vi "TIO Access Module Run.vi"(5 "Notification Prefix":string="Default", 8 "error in (no error)":errorcluster, 11 "TS Connection":T1={"Type"=enum."TCP", "Serial"="serial:///dev/cu.usbserial-00000", "TCP"=refnum, "Timeout"=500}) -> ()   [LabVIEW 2017]
uses:
  <vilib>/Utility/error.llb/Clear Errors.vi
  <instrlib>/tio-labview/TIO Library/Socket/TIO Stream Write.vi
  <instrlib>/tio-labview/TIO Library/RPC/RPC Helpers/TIO RPC Form Request.vi
  <instrlib>/tio-labview/TIO Library/Socket/Helpers/TIO SLIP Serial Write.vi
  <instrlib>/tio-labview/TIO Library/Socket/Helpers/TIO Form Packet.vi
  <instrlib>/tio-labview/TIO Library/Socket/Helpers/TIO SLIP Encode.vi
  <instrlib>/tio-labview/TIO Library/Socket/Helpers/TIO Serial Checksum CRC32.vi
panel:
  out "Kill":bool=TRUE
  out "Last Log":string
  out "Last PUB":string
  out "Last REQ":string
  # "TIO Proxy Run"
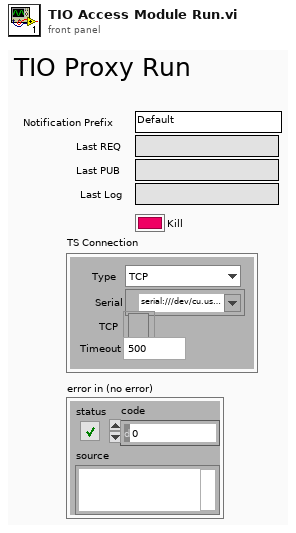
[diagram p1: front panel]
types:
  T1 = cluster{"Type":enum16{"TCP", "Serial"}, "Serial":refnum<visa-resource-name>, "TCP":refnum<k5>, "Timeout":u32}
  T2 = enum16{"big-endian, network order", "native, host order", "little-endian"}
  T3 = cluster{"Stream Description":cluster{"Stream ID":u16, "Data Type":u8, "Channels":u8, "Restart ID":u16, "Start timestamp (s)":dbl, "Sample counter":u64, "Period (s)":dbl, "Flags":u8, "Timestamp type":u8, "Name":string, "Last sample number":u64, "Last Restart ID":u16, "Version":u16, "Sample Size":u16}, "Sample #":u32, "Raw Data":string}
  T4 = cluster{"Stream ID":u16, "Data Type":u8, "Channels":u8, "Restart ID":u16, "Start timestamp (s)":dbl, "Sample counter":u64, "Period (s)":dbl, "Flags":u8, "Timestamp type":u8, "Name":string, "Last sample number":u64, "Last Restart ID":u16, "Version":u16, "Sample Size":u16}
  T5 = cluster{"Stream ID":u16, "Data Type":u8, "Channels":u8, "Restart ID":u16, "Start timestamp (s)":dbl, "Sample counter":u64, "Period (s)":dbl, "Flags":u8, "Timestamp type":u8, "Name":string, "Last sample number":u64, "Last Restart ID":u16, "Version":u16, "Sample Size":u16}[]
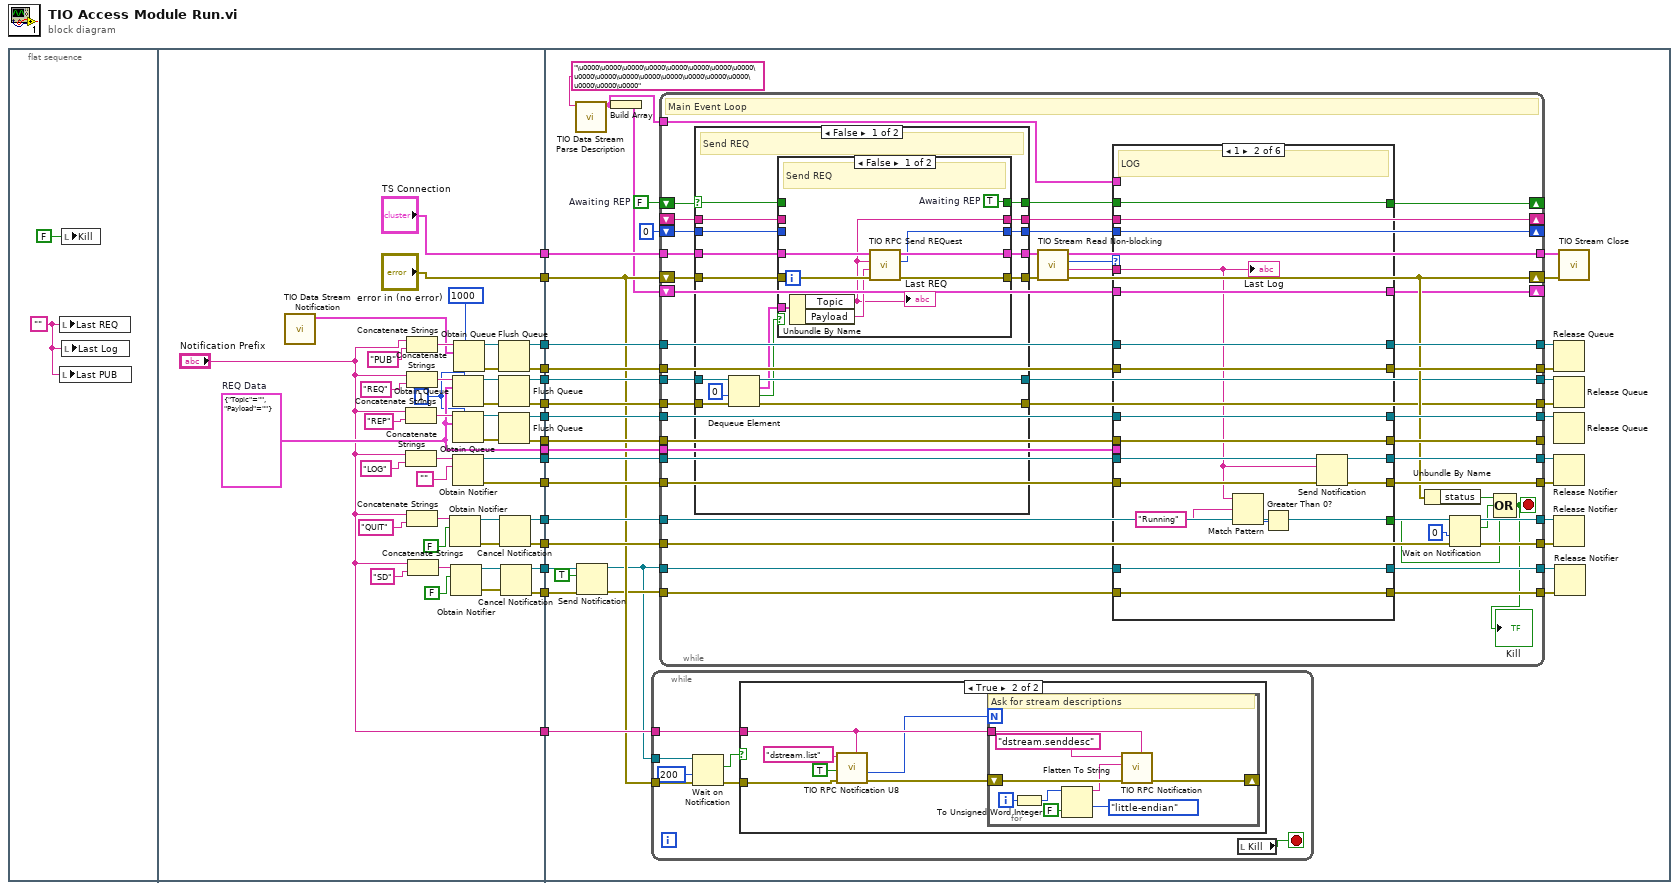
[diagram p0: block diagram]
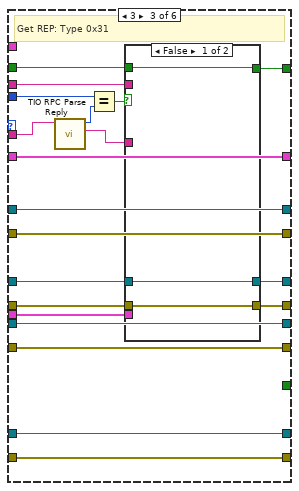
[diagram p4: hidden frame]
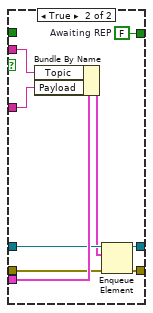
[diagram p5: hidden frame]
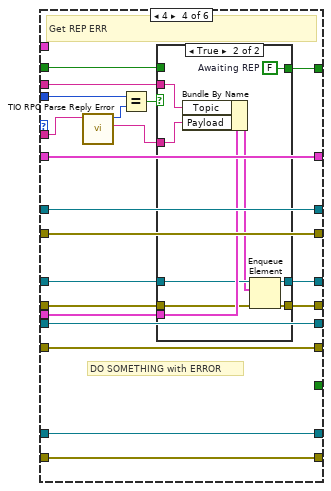
[diagram p6: hidden frame]
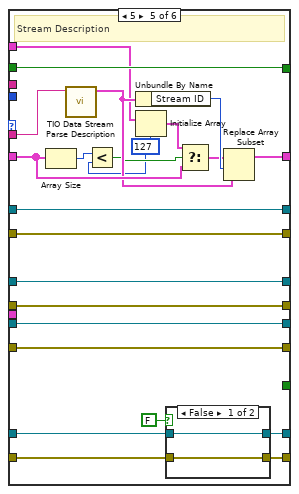
[diagram p8: hidden frame]
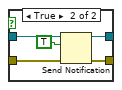
[diagram p9: hidden frame]
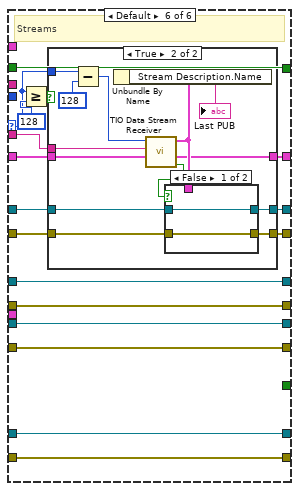
[diagram p10: hidden frame]
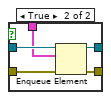
[diagram p12: hidden frame]
diagram:
  n1 = flat-sequence {
    tunnel: [w49] -> w16
    tunnel: ["Notification Prefix"] -> w15
    tunnel: ["TS Connection"] -> w14
    tunnel: ["error in (no error)"] -> w13
    tunnel: [w48] -> w12
    tunnel: [w38] -> w11
    tunnel: [w36] -> w10
    tunnel: [w35] -> w9
    tunnel: [w34] -> w8
    tunnel: [w40] -> w7
    tunnel: [w30] -> w6
    tunnel: [w29] -> w5
    tunnel: [w47] -> w4
    tunnel: [w46] -> w3
    tunnel: [w22] -> w2
    tunnel: [w21] -> w1
    tunnel: w16 -> [w92]
    tunnel: w15 -> [w80]
    tunnel: w14 -> [w91]
    tunnel: w13 -> [w79]
    tunnel: w12 -> [w90]
    tunnel: w11 -> [w89]
    tunnel: w10 -> [w88]
    tunnel: w9 -> [w87]
    tunnel: w8 -> [w86]
    tunnel: w7 -> [w85]
    tunnel: w6 -> [w84]
    tunnel: w5 -> [w83]
    tunnel: w4 -> [w82]
    tunnel: w3 -> [w81]
    tunnel: w2 -> [w71]
    tunnel: w1 -> [w70]
    frame #0 {
      w18 = ""
      n2 = local write "Last REQ"(w18) -> ()
      n3 = local write "Last PUB"(w18) -> ()
      n4 = local write "Kill"(FALSE ("Running")) -> ()
      n5 = local write "Last Log"(w18) -> ()
    }
    frame #1 {
      w33 = 1 ("max queue size (-1, unlimited)")
      w40 = cluster{"Topic":string, "Payload":string} {"Topic"="", "Payload"=""}  # REQ Data
      n6 = call <instrlib>:"TIO Data Stream Notification.vi"() -> ("Data Stream Notification"=w45:T3)  [unwired: 11 in]
      n7 = Concatenate Strings("Notification Prefix", "REP" ("name (unnamed)")) -> (w41:string)
      n8 = Concatenate Strings("Notification Prefix", "LOG" ("name (unnamed)")) -> (w32:string)
      n9 = Concatenate Strings("Notification Prefix", "PUB" ("name (unnamed)")) -> (w56:string)
      n10 = Concatenate Strings("Notification Prefix", "REQ" ("name (unnamed)")) -> (w42:string)
      n11 = Concatenate Strings("Notification Prefix", "QUIT" ("name (unnamed)")) -> (w52:string)
      n12 = Concatenate Strings("Notification Prefix", "SD" ("name (unnamed)")) -> (w26:string)
      n13 = Obtain Notifier(name (unnamed)=w52, notification data type=FALSE ("Connected")) -> (notifier out=w59:refnum<notifier>, error out=w60:errorcluster)  [unwired: 2 in, 1 out]
      n14 = Obtain Notifier(name (unnamed)=w26, notification data type=FALSE ("Connected")) -> (notifier out=w25:refnum<notifier>, error out=w24:errorcluster)  [unwired: 2 in, 1 out]
      n15 = Obtain Queue(max queue size (-1, unlimited)=w33, name (unnamed)=w42, element data type=w40) -> (queue out=w39:refnum<queue>, error out=w37:errorcluster)  [unwired: 2 in, 1 out]
      n16 = Obtain Queue(max queue size (-1, unlimited)=w33, name (unnamed)=w41, element data type=w40) -> (queue out=w44:refnum<queue>, error out=w43:errorcluster)  [unwired: 2 in, 1 out]
      n17 = Obtain Notifier(name (unnamed)=w32, notification data type="") -> (notifier out=w30:refnum<notifier>, error out=w29:errorcluster)  [unwired: 2 in, 1 out]
      n18 = Obtain Queue(max queue size (-1, unlimited)=1000, name (unnamed)=w56, element data type=w45) -> (queue out=w57:refnum<queue>, error out=w58:errorcluster)  [unwired: 2 in, 1 out]
      n19 = Flush Queue(queue=w57, error in (no error)=w58) -> (queue out=w49:refnum<queue>, error out=w48:errorcluster)  [unwired: 1 out]
      n20 = Flush Queue(queue=w39, error in (no error)=w37) -> (queue out=w38:refnum<queue>, error out=w36:errorcluster)  [unwired: 1 out]
      n21 = Flush Queue(queue=w44, error in (no error)=w43) -> (queue out=w35:refnum<queue>, error out=w34:errorcluster)  [unwired: 1 out]
      n22 = Cancel Notification(0:w59, 3:w60) -> (8:w47:refnum<notifier>, 11:w46:errorcluster)  [unwired: 1 out]
      n23 = Cancel Notification(0:w25, 3:w24) -> (8:w22:refnum<notifier>, 11:w21:errorcluster)  [unwired: 1 out]
    }
    frame #2 {
      w72 = FALSE  # Awaiting REP
      n24 = call <instrlib>:"TIO Data Stream Parse Description.vi"("Raw Stream Description"="\u0000\u0000\u0000\u0000\u0000\u0000\u0000\u0000\u0000\u0000\u0000\u0000\u0000\u0000\u0000\u0000\u0000\u0000\u0000") -> ("Stream Description"=w63:T4)  [unwired: 10 in]
      n25 = Send Notification(notification=TRUE, notifier=w71, error in (no error)=w70) -> (notifier out=w66:refnum<notifier>, error out=w69:errorcluster)
      n26 = Build Array(w63) -> (w78:T5)
      n27 = while {
        tunnel: w80 -> [w106]
        tunnel: w79 -> [w105]
        tunnel: w66 -> [w103]
        stop <- w102 stop-if-true
        n28 = Wait on Notification(notifier=w103, timeout in ms (-1)=200, error in (no error)=w105) -> (notification=w100:bool, error out=w104:errorcluster)  [unwired: 1 in, 2 out]
        n29 = case shown="True" w100 {
          tunnel: w106 -> [_ w112]
          tunnel: w104 -> [_ w107]
          frame False {
          }
          frame True {
            n30 = call <instrlib>:"TIO RPC Notification U8.vi"("Notification Prefix"=w112, "error in (no error)"=w107, "Read"=TRUE, "String"="dstream.list" ("Topic")) -> ("error out"=w109:errorcluster, "U8"=w110:u8)  [unwired: 4 in, 1 out]
            n31 = for {
              N: w110 -> [_]
              shift-right: [w120] -> _
              shift-left: w109 -> [w121]
              tunnel: w112 -> [w118]
              i -> [w117]
              # "Ask for stream descriptions"
              n32 = To Unsigned Word Integer(number=w117) -> (unsigned 16bit integer=w116:u16)
              n33 = Flatten To String(anything=w116, prepend array or string size? (T)=FALSE, byte order (0:big-endian, network order)=T2."little-endian") -> (data string=w113:string)  [unwired: 1 in, 2 out]
              n34 = call <instrlib>:"TIO RPC Notification.vi"("Notification Prefix"=w118, "error in (no error)"=w121, "Payload"=w113, "Topic"="dstream.senddesc") -> ("error out"=w120:errorcluster)  [unwired: 4 in, 2 out]
            }
          }
        }
        n35 = local read "Kill"() -> (w102:bool)
      }
      n36 = while {
        shift-right: [w139] -> w98
        shift-left: w79 -> [w163]
        tunnel: w89 -> [w135]
        tunnel: [w134] -> w73
        tunnel: w92 -> [w169]
        tunnel: w85 -> [w168]
        tunnel: [w167] -> w99
        tunnel: w87 -> [w166]
        tunnel: [w165] -> w74
        tunnel: w91 -> [w164]
        tunnel: [w161] -> w97
        tunnel: [w155] -> w96
        tunnel: [w154] -> w95
        tunnel: w82 -> [w153]
        tunnel: w81 -> [w152]
        tunnel: w88 -> [w133]
        tunnel: [w132] -> w77
        tunnel: w86 -> [w151]
        tunnel: [w150] -> _
        tunnel: w90 -> [w149]
        tunnel: [w148] -> w94
        shift-right: [w147] -> _
        shift-left: u16 0 ("Request ID") -> [w146]
        shift-right: [w144] -> _
        shift-left: _ -> [w145]
        tunnel: w84 -> [w140]
        tunnel: [w141] -> w75
        tunnel: w83 -> [w142]
        tunnel: [w143] -> w76
        shift-right: [w137] -> _
        shift-left: w78 -> [w136]
        shift-right: [w130] -> _
        shift-left: w72 -> [w129]
        tunnel: w66 -> [w128]
        tunnel: w69 -> [w127]
        tunnel: [w126] -> w68
        tunnel: [w125] -> w67
        tunnel: w63 -> [w123]
        stop <- w124 stop-if-true
        # "Main Event Loop"
        n37 = case shown="False" w129 {
          selector: w129 -> [w330 w367]
          tunnel: w164 -> [w346 w364]
          tunnel: w163 -> [w345 w363]
          tunnel: [w344 w364] -> w160
          tunnel: [w343 w363] -> w159
          tunnel: [w342 w365] -> w147
          tunnel: w146 -> [w341 w365]
          tunnel: w145 -> [w340 w366]
          tunnel: [w339 w366] -> w144
          tunnel: w135 -> [w338 w362]
          tunnel: [w337 w362] -> w134
          tunnel: w133 -> [w336 w361]
          tunnel: [w335 w361] -> w132
          tunnel: [w331 w367] -> w131
          frame False {
            # "Send REQ"
            n38 = Dequeue Element(queue=w338, timeout in ms (-1)=0, error in (no error)=w336) -> (queue out=w337:refnum<queue>, element=w333:cluster{"Topic":string, "Payload":string}, timed out?=w332:bool, error out=w335:errorcluster)
            n39 = case shown="False" w332 {
              tunnel: w345 -> [w355 w360]
              tunnel: [w354 w360] -> w343
              tunnel: [w353 w359] -> w344
              tunnel: w346 -> [w352 w359]
              tunnel: w333 -> [w350 _]
              tunnel: [w349 w358] -> w342
              tunnel: w341 -> [_ w358]
              tunnel: [w348 w357] -> w339
              tunnel: w340 -> [_ w357]
              tunnel: w330 -> [_ w356]
              tunnel: [w347 w356] -> w331
              frame False {
                w347 = TRUE  # Awaiting REP
                # "Send REQ"
                n40 = Unbundle By Name(w350) -> ("Topic"=w348:string, "Payload"=w351:string)
                "Last REQ" <- w348
                n41 = call <instrlib>:"TIO RPC Send REQuest.vi"("error in (no error)"=w355, "Payload"=w351, "Topic"=w348, "TS Connection"=w352) -> ("error out"=w354:errorcluster, "Request ID"=w349:u16, "TS Connection"=w353:T1)  [unwired: 5 in]
              }
              frame True {
                # "REQ Notification timeout"
              }
            }
          }
          frame True {
            # "Awaiting REP"
          }
        }
        n42 = call <instrlib>:"TIO Stream Read Non-blocking.vi"("error in (no error)"=w159, "TS Connection"=w160) -> ("error out"=w139:errorcluster, "Payload"=w157:string, "Type"=w158:u16, "TS Connection"=w161:T1)  [unwired: 6 in]
        n43 = case shown="1" w158 {
          selector: w158 -> [_ _ _ _ _ w294]
          tunnel: w169 -> [w179 w195 w213 w245 w282 w306]
          tunnel: w168 -> [_ _ w215 w247 _ _]
          tunnel: w157 -> [_ w183 w211 w230 w276 w298]
          tunnel: [w179 w195 w213 w245 w282 w305] -> w167
          tunnel: w166 -> [w178 w194 w214 w246 w280 w304]
          tunnel: [w178 w194 w212 w244 w280 w304] -> w165
          tunnel: w151 -> [w177 w192 w209 w243 w279 w301]
          tunnel: [w177 w192 w208 w242 w279 w301] -> w150
          tunnel: w149 -> [w176 w193 w207 w241 w281 w303]
          tunnel: [w176 w193 w207 w241 w281 w302] -> w148
          tunnel: w147 -> [_ _ w204 w239 _ _]
          tunnel: w144 -> [_ _ w206 w240 _ _]
          tunnel: w140 -> [w175 w190 w202 w237 w278 w300]
          tunnel: [w175 w188 w202 w237 w278 w300] -> w141
          tunnel: w142 -> [w174 w189 w201 w236 w277 w299]
          tunnel: [w174 w187 w201 w236 w277 w299] -> w143
          tunnel: [w173 w191 w200 w235 w274 w296] -> w137
          tunnel: w136 -> [w173 w191 w200 w235 w273 w297]
          tunnel: w131 -> [w172 w186 w199 w234 w266 w292]
          tunnel: [w172 w186 w198 w233 w266 w292] -> w130
          tunnel: w128 -> [w171 w185 w197 w232 w265 w291]
          tunnel: w127 -> [w170 w184 w196 w231 w263 w290]
          tunnel: [w171 w185 w197 w232 w264 w291] -> w126
          tunnel: [w170 w184 w196 w231 w262 w290] -> w125
          tunnel: w123 -> [_ _ _ _ w260 _]
          tunnel: [_ w180 _ _ _ _] -> w122
          frame 0 {
          }
          frame 1 {
            # "LOG"
            n44 = Match Pattern(string=w183, regular expression="Running" ("string")) -> (offset past match=w181:i32)  [unwired: 1 in, 3 out]
            n45 = Greater Than 0?(x=w181) -> (x > 0?=w180:bool)
            n46 = Send Notification(notification=w183, notifier=w190, error in (no error)=w189) -> (notifier out=w188:refnum<notifier>, error out=w187:errorcluster)
            "Last Log" <- w183
          }
          frame 3 {
            # "Get REP: Type 0x31"
            n47 = call <instrlib>:"TIO RPC Parse Reply.vi"("Payload"=w211) -> ("Payload"=w210:string, "Request ID"=w205:u16)  [unwired: 9 in]
            n48 = Equal?(x=w204, y=w205) -> (x = y?=w203:bool)
            n49 = case shown="False" w203 {
              tunnel: w215 -> [_ w227]
              tunnel: w214 -> [w218 w224]
              tunnel: [w218 w223] -> w212
              tunnel: w210 -> [_ w226]
              tunnel: w209 -> [w217 w222]
              tunnel: [w217 w221] -> w208
              tunnel: w206 -> [_ w225]
              tunnel: w199 -> [w216 _]
              tunnel: [w216 w219] -> w198
              frame False {
              }
              frame True {
                w219 = FALSE  # Awaiting REP
                n50 = Bundle By Name(cluster=w227, "Topic"=w225, "Payload"=w226) -> (w220:cluster{"Topic":string, "Payload":string})
                n51 = Enqueue Element(queue=w224, element=w220, error in (no error)=w222) -> (queue out=w223:refnum<queue>, error out=w221:errorcluster)  [unwired: 1 in, 1 out]
              }
            }
          }
          frame 4 {
            # "DO SOMETHING with ERROR"
            # "Get REP ERR"
            n52 = call <instrlib>:"TIO RPC Parse Reply Error.vi"("Payload"=w230) -> ("Payload"=w228:string, "Request ID"=w229:u16)  [unwired: 8 in, 1 out]
            n53 = Equal?(x=w239, y=w229) -> (x = y?=w238:bool)
            n54 = case shown="True" w238 {
              tunnel: w247 -> [_ w259]
              tunnel: w246 -> [w250 w256]
              tunnel: [w250 w255] -> w244
              tunnel: w228 -> [_ w258]
              tunnel: w243 -> [w249 w254]
              tunnel: [w249 w253] -> w242
              tunnel: w240 -> [_ w257]
              tunnel: w234 -> [w248 _]
              tunnel: [w248 w251] -> w233
              frame False {
              }
              frame True {
                w251 = FALSE  # Awaiting REP
                n55 = Bundle By Name(cluster=w259, "Topic"=w257, "Payload"=w258) -> (w252:cluster{"Topic":string, "Payload":string})
                n56 = Enqueue Element(queue=w256, element=w252, error in (no error)=w254) -> (queue out=w255:refnum<queue>, error out=w253:errorcluster)  [unwired: 1 in, 1 out]
              }
            }
          }
          frame 5 {
            w267 = 127 ("dimension size")
            # "Stream Description"
            n57 = Array Size(array=w273) -> (size(s)=w269:i32)
            n58 = call <instrlib>:"TIO Data Stream Parse Description.vi"("Raw Stream Description"=w276) -> ("Stream Description"=w270:T4)  [unwired: 10 in]
            n59 = Less?(x=w269, y=w267) -> (x < y?=w268:bool)
            n60 = Unbundle By Name(w270) -> ("Stream ID"=w275:u16)
            n61 = Initialize Array(w260, w267) -> (w272:T5)
            n62 = case shown="False" FALSE {
              tunnel: w265 -> [w284 w289]
              tunnel: [w284 w288] -> w264
              tunnel: w263 -> [w283 w287]
              tunnel: [w283 w286] -> w262
              frame False {
              }
              frame True {
                n63 = Send Notification(notification=TRUE, notifier=w289, error in (no error)=w287) -> (notifier out=w288:refnum<notifier>, error out=w286:errorcluster)
              }
            }
            n64 = Select(t=w272, s=w268, f=w273) -> (s? t:f=w271:T5)
            n65 = Replace Array Subset(array=w271, new element=w270, index=w275) -> (w274:T5)
          }
          frame Default {
            # "Streams"
            n66 = Greater Or Equal?(x=w294, y=u16 128) -> (x >= y?=w293:bool)
            n67 = case shown="True" w293 {
              tunnel: w306 -> [w308 w322]
              tunnel: [w308 w321] -> w305
              tunnel: w303 -> [w307 w320]
              tunnel: [w307 w319] -> w302
              tunnel: w298 -> [_ w318]
              tunnel: w297 -> [w309 w312]
              tunnel: [w309 w311] -> w296
              tunnel: w294 -> [_ w314]
              frame False {
              }
              frame True {
                n68 = Subtract(x=w314, y=u16 128) -> (x-y=w316:u16)
                n69 = call <instrlib>:"TIO Data Stream Receiver.vi"("Stream Info In"=w312, "Raw Stream Data"=w318, "Stream ID"=w316) -> ("Known Stream"=w310:bool, "Stream Info Out"=w311:T5, "Data Stream Notification"=w315:T3)  [unwired: 6 in]
                n70 = Unbundle By Name(w315) -> ("Stream Description.Name"=→"Last PUB":string)
                n71 = case shown="False" w310 {
                  tunnel: w322 -> [w324 w329]
                  tunnel: [w324 w328] -> w321
                  tunnel: w320 -> [w323 w327]
                  tunnel: [w323 w326] -> w319
                  tunnel: w315 -> [_ w325]
                  frame False {
                  }
                  frame True {
                    n72 = Enqueue Element(queue=w329, element=w325, error in (no error)=w327) -> (queue out=w328:refnum<queue>, error out=w326:errorcluster)  [unwired: 1 in, 1 out]
                  }
                }
              }
            }
          }
        }
        n73 = Unbundle By Name(w139) -> ("status"=w162:bool)
        n74 = Wait on Notification(notifier=w153, timeout in ms (-1)=0, error in (no error)=w152) -> (notifier out=w155:refnum<notifier>, notification=w138:bool, error out=w154:errorcluster)  [unwired: 1 in, 1 out]
        n75 = Compound Arithmetic op=OR(w162, w138, w122) -> (w124:bool)
        "Kill" <- w124
      }
      n76 = Release Queue(queue=w99, error in (no error)=w94) -> ()  [unwired: 1 in, 3 out]
      n77 = Release Queue(queue=w73, error in (no error)=w77) -> ()  [unwired: 1 in, 3 out]
      n78 = Release Queue(queue=w74) -> ()  [unwired: 2 in, 3 out]
      n79 = Release Notifier(notifier=w75, error in (no error)=w76) -> ()  [unwired: 1 in, 3 out]
      n80 = Release Notifier(notifier=w96, error in (no error)=w95) -> ()  [unwired: 1 in, 3 out]
      n81 = Release Notifier(notifier=w68, error in (no error)=w67) -> ()  [unwired: 1 in, 3 out]
      n82 = call <instrlib>:"TIO Stream Close.vi"("error in (no error)"=w98, "TS Connection"=w97) -> ()  [unwired: 10 in]
    }
  }
